vi "SunyeeTestMain.vi"() -> ()   [LabVIEW 2018]
uses:
  <vilib>/Utility/error.llb/DialogType.ctl
  <vilib>/DAQmx/write.llb/DAQmx Write (Digital 1D Wfm NChan NSamp).vi
  <vilib>/DAQmx/write.llb/DAQmx Write (Analog 1D Wfm NChan NSamp).vi
  <vilib>/DAQmx/create/channels.llb/DAQmx Create Channel (AO-Voltage-Basic).vi
  <vilib>/DAQmx/configure/timing.llb/DAQmx Timing (Sample Clock).vi
  <vilib>/DAQmx/create/channels.llb/DAQmx Create Channel (DO-Digital Output).vi
  <vilib>/DAQmx/configure/trigger.llb/DAQmx Start Trigger (Digital Edge).vi
  <vilib>/DAQmx/configure/trigger.llb/DAQmx Start Trigger (Time).vi
  <vilib>/Waveform/WDTOps.llb/WDT Append Waveforms DBL.vi
  <vilib>/DAQmx/miscellaneous.llb/DAQmx Fill In Error Info.vi
  <vilib>/Waveform/DWDTOps.llb/DWDT Uncompress Digital.vi
  <resource>/objmgr/daqmx.rc
panel:
  out "Digital Waveform Graph2":digitalwaveform(graph)
  out "Digital Waveform Graph1":digitalwaveform(graph)
  out "AO Actual Sample Rate":dbl=1000.0 format="%0.2f"
  out "Digital Waveform Graph":digitalwaveform[](graph)
  in  "lines":tag="PXI1Slot4_2/port0/line0:1"
  in  "error in":errorcluster
  in  "Trigger Type":T1(tab)
  in  "Edge":i32(ring)=10280 items=["Rising"=10280, "Falling"=10171]
  in  "Digital Trigger Source":tag="PFI1"
  in  "When":timestamp
  in  "Select Time\nManually":bool
  out "DO Actual Sample Rate":dbl=1000.0 format="%0.2f"
  out "Waveform Graph2":waveform(dbl)(graph)
  out "Waveform Graph 1":waveform(dbl)(graph)
  out "Waveform Graph":waveform(dbl)[](graph)
  in  "Stop":bool
  in  "Physical Channel(s)":tag="PXI1Slot4_2/ao0:7"
  # "To configure and use a start trigger you must have the necessary tab selected above.  Not all hardware supports triggering--refer to your device documentation for more info."
  # "If time is not manually set, task will begin after 10 seconds"
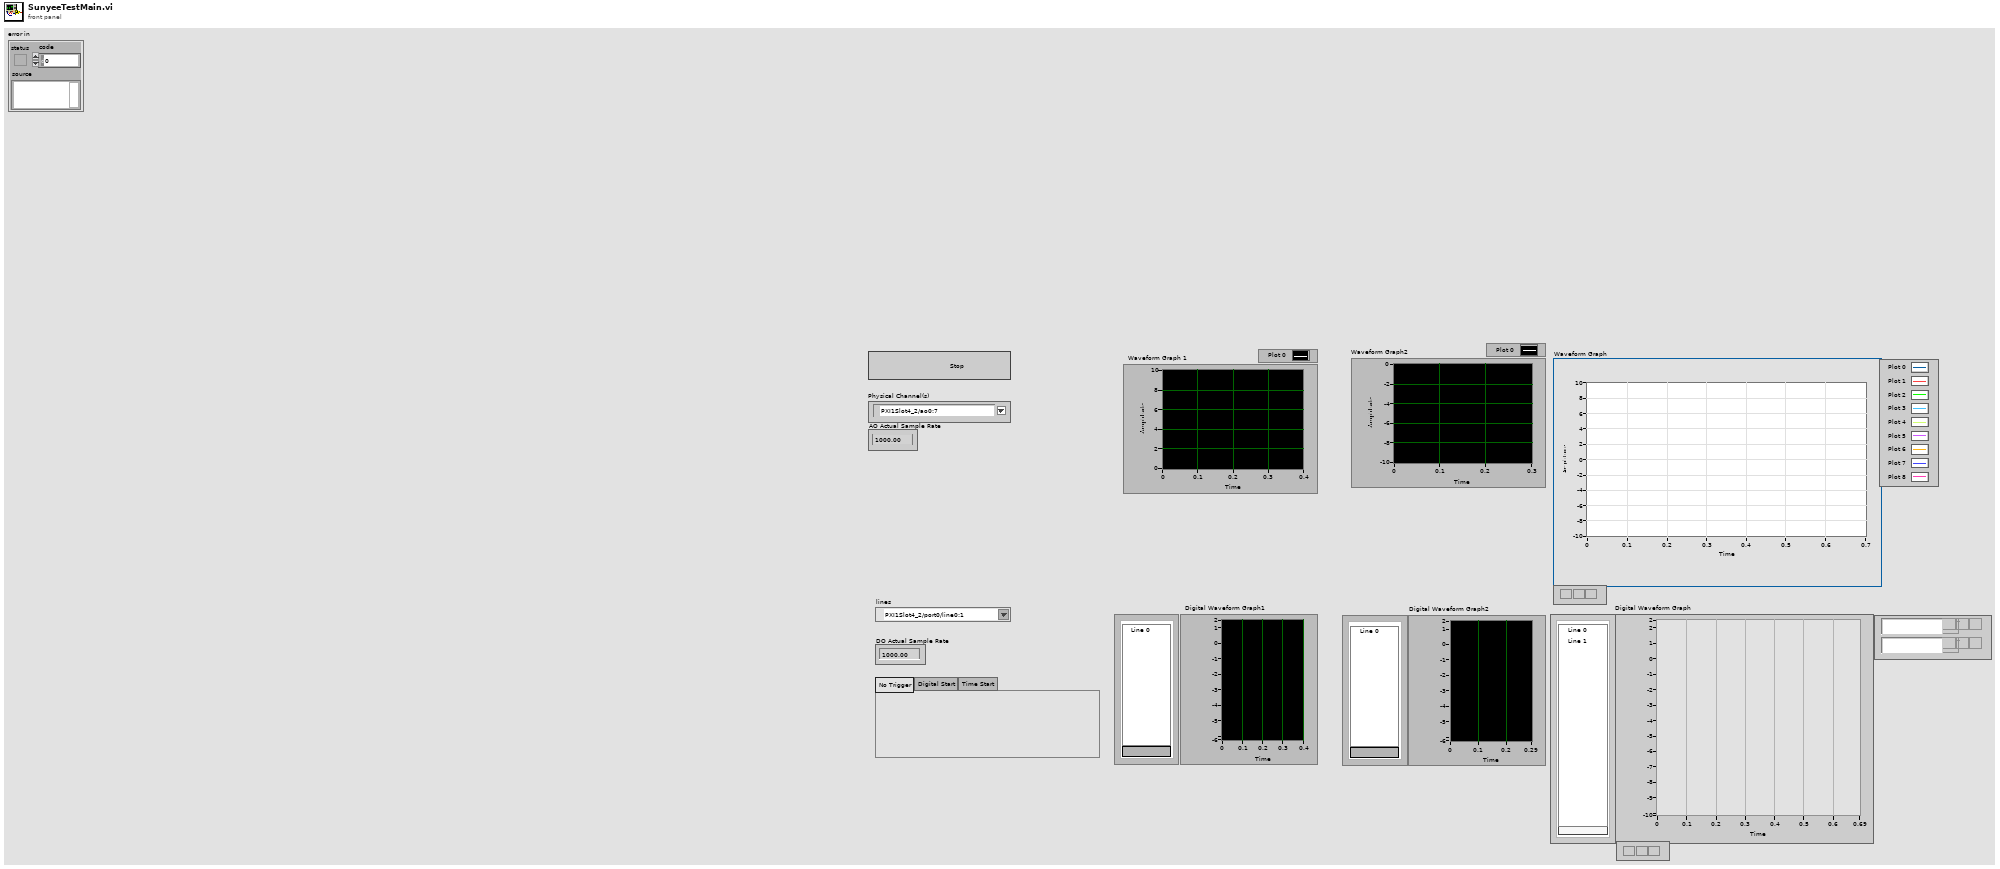
[diagram p1: front panel]
types:
  T1 = enum32{"No Trigger", "Digital Start", "Time Start"}
  T2 = typedef "DialogType.ctl" = u16
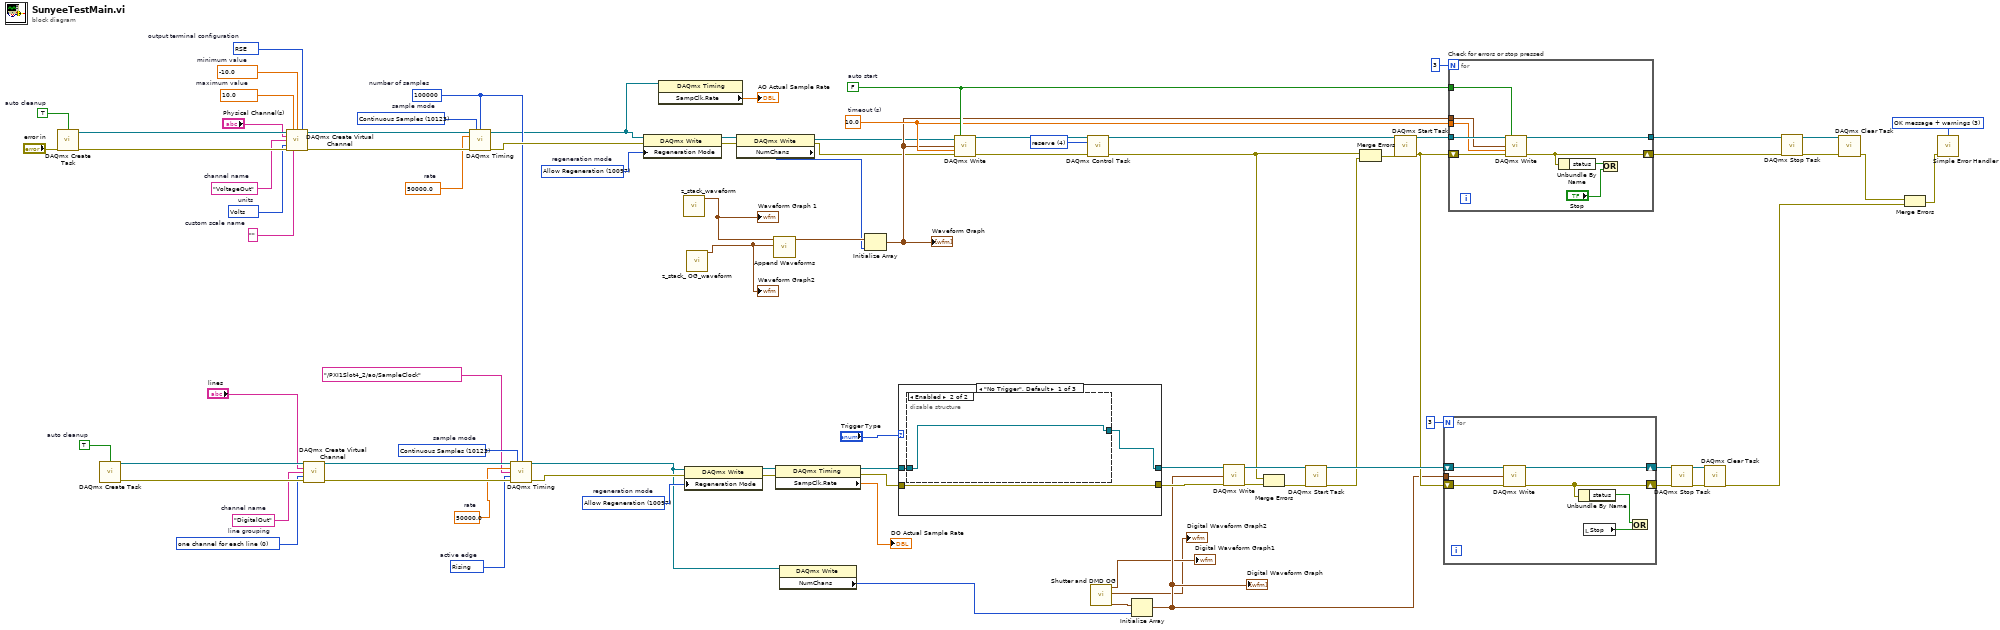
[diagram p0: block diagram]
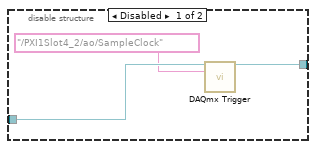
[diagram p2: hidden frame]
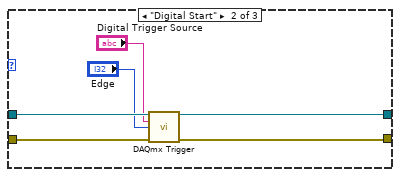
[diagram p3: hidden frame]
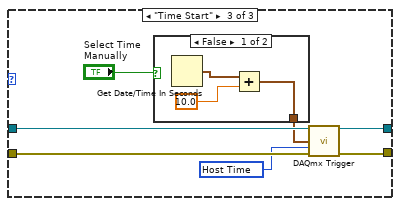
[diagram p4: hidden frame]
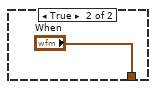
[diagram p5: hidden frame]
diagram:
  w33 = T2 3 items=["no dialog", "OK message", "continue or stop message", "OK message + warnings", "continue/stop + warnings"] ("type of dialog (OK msg:1)")
  w35 = 10097 items=["Allow Regeneration"=10097, "Do Not Allow Regeneration"=10158]  # regeneration mode
  w36 = 10123 items=["Finite Samples"=10178, "Continuous Samples"=10123, "Hardware Timed Single Point"=12522]  # sample mode
  w21 = 100000  # number of samples
  w37 = 50000.0  # rate
  w40 = 10083 items=["Default"=-1, "RSE"=10083, "Differential"=10106, "Pseudodifferential"=12529]  # output terminal configuration
  w41 = 10348 items=["Volts"=10348, "From Custom Scale"=10065]  # units
  w42 = "VoltageOut"  # channel name
  w44 = ""  # custom scale name
  w45 = -10.0  # minimum value
  w46 = 10.0  # maximum value
  w48 = TRUE  # auto cleanup
  w55 = 4 items=["verify"=2, "reserve"=4, "commit"=3, "unreserve"=5, "abort"=6] ("action")
  w62 = 10097 items=["Allow Regeneration"=10097, "Do Not Allow Regeneration"=10158]  # regeneration mode
  w63 = 10123 items=["Finite Samples"=10178, "Continuous Samples"=10123, "Hardware Timed Single Point"=12522]  # sample mode
  w61 = 50000.0  # rate
  w64 = 10280 items=["Rising"=10280, "Falling"=10171]  # active edge
  w69 = 0 items=["one channel for each line", "one channel for all lines"]  # line grouping
  w68 = "DigitalOut"  # channel name
  w71 = TRUE  # auto cleanup
  w84 = 10.0  # timeout (s)
  w85 = FALSE  # auto start
  n1 = call <vilib>:"DAQmx Create Task.vi"("auto cleanup"=w48, "error in"="error in") -> ("task out"=w47:refnum<k21>, "error out"=w49:errorcluster)  [unwired: 12 in]
  n2 = call <vilib>:"DAQmx Create Task.vi"("auto cleanup"=w71) -> ("task out"=w70:refnum<k21>, "error out"=w72:errorcluster)  [unwired: 13 in]
  n3 = call-poly <vilib>:"DAQmx Create Virtual Channel.vi"("task in"=w47, "maximum value"=w46, "minimum value"=w45, "output terminal configuration"=w40, "physical channels"="Physical Channel(s)", "name to assign"=w42, "units"=w41, "error in"=w49, "custom scale name"=w44) -> ("task out"=w38:refnum<k21>, "error out"=w43:errorcluster)  [unwired: 5 in]
  n4 = call-poly <vilib>:"DAQmx Create Virtual Channel.vi"("task in"=w70, "lines"="lines", "name to assign"=w68, "line grouping"=w69, "error in"=w72) -> ("task out"=w65:refnum<k21>, "error out"=w67:errorcluster)  [unwired: 9 in]
  n5 = call-poly <vilib>:"DAQmx Timing.vi"("task/channels in"=w38, "sample mode"=w36, "samples per channel"=w21, "rate"=w37, "error in"=w43) -> ("task out"=w14:refnum<k21>, "error out"=w39:errorcluster)  [unwired: 9 in]
  n6 = call-poly <vilib>:"DAQmx Timing.vi"("task/channels in"=w65, "sample mode"=w63, "samples per channel"=w21, "rate"=w61, "source"=tag "/PXI1Slot4_2/ao/SampleClock", "active edge"=w64, "error in"=w67) -> ("task out"=w2:refnum<k21>, "error out"=w66:errorcluster)  [unwired: 7 in]
  n7 = property class="DAQmx Write"(reference=w14, error in=w39, "Regeneration Mode"=w35) -> (reference out=w19:refnum<k21>, error out=w18:errorcluster)
  n8 = property class="DAQmx Timing"(reference=w14) -> ("SampClk.Rate"=→"AO Actual Sample Rate":dbl)  [unwired: 1 in, 2 out]
  n9 = call "z_stack_waveform.vi"() -> ("waveform out"=w29:waveform(dbl))  [unwired: 9 in, 2 out]
  "Waveform Graph 1" <- w29
  n10 = property class="DAQmx Write"(reference=w2, error in=w66, "Regeneration Mode"=w62) -> (reference out=w59:refnum<k21>, error out=w3:errorcluster)
  n11 = call "z_stack_ OG_waveform.vi"() -> ("waveform out"=w28:waveform(dbl))  [unwired: 15 in, 4 out]
  "Waveform Graph2" <- w28
  n12 = property class="DAQmx Write"(reference=w19, error in=w18) -> (reference out=w17:refnum<k21>, error out=w16:errorcluster, "NumChans"=w15:u32)
  n13 = call-poly <vilib>:"Append Waveforms.vi"("waveform B"=w28, "waveform A"=w29) -> ("waveform out"=w34:waveform(dbl))  [unwired: 8 in, 1 out]
  n14 = property class="DAQmx Timing"(reference=w59, error in=w3) -> (reference out=w81:refnum<k21>, error out=w80:errorcluster, "SampClk.Rate"=→"DO Actual Sample Rate":dbl)
  n15 = property class="DAQmx Write"(reference=w2) -> ("NumChans"=w1:u32)  [unwired: 1 in, 2 out]
  n16 = Initialize Array(w34, w15) -> (w27:waveform(dbl)[])
  "Waveform Graph" <- w27
  n17 = case shown="\"No Trigger\", Default" "Trigger Type" {
    tunnel: w81 -> [w88 w99 w106]
    tunnel: w80 -> [w89 w98 w105]
    tunnel: [w87 w97 w104] -> w74
    tunnel: [w89 w96 w103] -> w73
    frame "No Trigger", Default {
      n18 = disable-structure shown="Enabled" {
        disable-tunnel: w88 -> [w92 w93]
        disable-tunnel: [w90 w93] -> w87
        frame Disabled {
          n19 = call-poly <vilib>:"DAQmx Trigger.vi"("task/channels in"=w92, "source"=tag "/PXI1Slot4_2/ao/SampleClock") -> ("task out"=w90:refnum<k21>)  [unwired: 12 in, 1 out]
        }
        frame Enabled {
        }
      }
    }
    frame "Digital Start" {
      n20 = call-poly <vilib>:"DAQmx Trigger.vi"("task/channels in"=w99, "source"="Digital Trigger Source", "edge"="Edge", "error in"=w98) -> ("task out"=w97:refnum<k21>, "error out"=w96:errorcluster)  [unwired: 10 in]
    }
    frame "Time Start" {
      w100 = 16126 items=["Host Time"=16126, "I/O Device Time"=16127] ("timescale")
      n21 = case shown="False" "Select Time\nManually" {
        tunnel: [w108 "When"] -> w101
        frame False {
          n22 = Get Date/Time In Seconds() -> (seconds since 1Jan1904=w109:timestamp)
          n23 = Add(x=w109, y=10.0) -> (x+y=w108:timestamp)
        }
        frame True {
        }
      }
      n24 = call-poly <vilib>:"DAQmx Trigger.vi"("task/channels in"=w106, "when"=w101, "timescale"=w100, "error in"=w105) -> ("task out"=w104:refnum<k21>, "error out"=w103:errorcluster)  [unwired: 10 in]
    }
  }
  n25 = call-poly <vilib>:"DAQmx Write.vi"("task/channels in"=w17, "auto start"=w85, "data"=w27, "timeout"=w84, "error in"=w16) -> ("task out"=w54:refnum<k21>, "error out"=w52:errorcluster)  [unwired: 8 in, 1 out]
  n26 = call <vilib>:"DAQmx Control Task.vi"("task/channels in"=w54, "action"=w55, "error in"=w52) -> ("task out"=w53:refnum<k21>, "error out"=w24:errorcluster)  [unwired: 11 in]
  n27 = call "Shutter and DMD OG.vi"() -> ("output waveform"=w57:digitalwaveform, "output waveform 2"=→"Digital Waveform Graph2":digitalwaveform, "output waveform1"=→"Digital Waveform Graph1":digitalwaveform)  [unwired: 8 in]
  n28 = Initialize Array(w57, w1) -> (w12:digitalwaveform[])
  "Digital Waveform Graph" <- w12
  n29 = call-poly <vilib>:"DAQmx Write.vi"("task/channels in"=w74, "data"=w12, "error in"=w73) -> ("task out"=w56:refnum<k21>, "error out"=w26:errorcluster)  [unwired: 10 in, 1 out]
  n30 = Merge Errors(w24, w26) -> (w25:errorcluster)
  n31 = call <vilib>:"DAQmx Start Task.vi"("task/channels in"=w56, "error in"=w25) -> ("task out"=w79:refnum<k21>, "error out"=w23:errorcluster)  [unwired: 12 in]
  n32 = Merge Errors(w24, w23) -> (w22:errorcluster)
  n33 = call <vilib>:"DAQmx Start Task.vi"("task/channels in"=w53, "error in"=w22) -> ("task out"=w86:refnum<k21>, "error out"=w51:errorcluster)  [unwired: 12 in]
  n34 = for {
    N: 3 -> [_]
    tunnel: w12 -> [w114]
    shift-right: [w116] -> w76
    shift-left: w79 -> [w117]
    shift-right: [w115] -> w75
    shift-left: w51 -> [w113]
    n35 = call-poly <vilib>:"DAQmx Write.vi"("task/channels in"=w117, "data"=w114, "error in"=w113) -> ("task out"=w116:refnum<k21>, "error out"=w115:errorcluster)  [unwired: 10 in, 1 out]
    n36 = Unbundle By Name(w115) -> ("status"=w112:bool)
    n37 = local read "Stop"() -> (w111:bool)
    n38 = Or(x=w112, y=w111) -> ()  [unwired: 1 out]
  }
  n39 = for "Check for errors or stop pressed" {
    N: 3 -> [_]
    tunnel: [w125] -> w30
    tunnel: w86 -> [w126]
    shift-right: [w122] -> w7
    shift-left: w51 -> [w124]
    tunnel: w85 -> [w121]
    tunnel: w27 -> [w120]
    tunnel: w84 -> [w119]
    n40 = call-poly <vilib>:"DAQmx Write.vi"("task/channels in"=w126, "auto start"=w121, "data"=w120, "timeout"=w119, "error in"=w124) -> ("task out"=w125:refnum<k21>, "error out"=w122:errorcluster)  [unwired: 8 in, 1 out]
    n41 = Unbundle By Name(w122) -> ("status"=w123:bool)
    n42 = Or(x=w123, y="Stop") -> ()  [unwired: 1 out]
  }
  n43 = call <vilib>:"DAQmx Stop Task.vi"("task/channels in"=w76, "error in"=w75) -> ("task out"=w78:refnum<k21>, "error out"=w77:errorcluster)  [unwired: 12 in]
  n44 = call <vilib>:"DAQmx Clear Task.vi"("task in"=w78, "error in"=w77) -> ("error out"=w5:errorcluster)  [unwired: 13 in]
  n45 = call <vilib>:"DAQmx Stop Task.vi"("task/channels in"=w30, "error in"=w7) -> ("task out"=w31:refnum<k21>, "error out"=w32:errorcluster)  [unwired: 12 in]
  n46 = call <vilib>:"DAQmx Clear Task.vi"("task in"=w31, "error in"=w32) -> ("error out"=w6:errorcluster)  [unwired: 13 in]
  n47 = Merge Errors(w6, w5) -> (w4:errorcluster)
  n48 = call <vilib>:"Simple Error Handler.vi"("type of dialog (OK msg:1)"=w33, "error in (no error)"=w4) -> ()  [unwired: 3 in, 5 out]
